vi "Angle Rotation.vi"   [LabVIEW 2020, in "NI_AAL_Angle.lvlib"]
doc: "Rotates the input angle counterclockwise.\n\nWire data to the angle input to determine the polymorphic instance to use or manually select the instance."
uses:
  <vilib>/Analysis/NI_AAL_Angle.lvlib
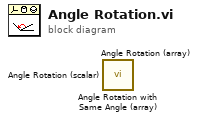
[diagram p0: block diagram]
diagram:
  n1 = call <vilib>:"Angle Rotation with Same Angle (array).vi"() -> ()  [unwired: 10 in, 2 out]
  n2 = call <vilib>:"Angle Rotation (array).vi"() -> ()  [unwired: 10 in, 2 out]
  n3 = call <vilib>:"Angle Rotation (scalar).vi"() -> ()  [unwired: 10 in, 2 out]
